vi "Register Image Event.vi"(8 "Error In":errorcluster, 10 "User Event":T1, 11 "Image Object":T2={"Device ID"=0, "Memeroy ID"=0, "Image Parameters"={"Channel Order"=enum."CL_LUMINANCE (Grayscale)", "Dimension"={"Depth"=1, "Height"=1, "Width"=1}, "Data Type"=enum."32f", "Offset"={"X"=0, "Y"=0, "Z"=0}}} {"Image Parameters"."Dimension"."Width" min=1; "Image Parameters"."Dimension"."Height" min=1; "Image Parameters"."Dimension"."Depth" min=1}) -> (0 "Error Out":errorcluster, 2 "User Event Out":T1, 3 "Memory Object Out":T2={"Device ID"=0, "Memeroy ID"=0, "Image Parameters"={"Channel Order"=enum."CL_LUMINANCE (Grayscale)", "Dimension"={"Depth"=1, "Height"=1, "Width"=1}, "Data Type"=enum."32f", "Offset"={"X"=0, "Y"=0, "Z"=0}}} {"Image Parameters"."Dimension"."Width" min=1; "Image Parameters"."Dimension"."Height" min=1; "Image Parameters"."Dimension"."Depth" min=1})   [LabVIEW 2012, in "OpenCLV x64.lvlib"]
doc: "Registers an image user event using a Boolean Labview User Event. Once an image has been registered with a Labview User Event, it can be read and written to asynchronously (non-blocking) to allow other tasks to be performed by the program including user inputs to the front panel.\n\nThis is useful when copying very large datasets to the device."
uses:
  OpenCLV x64.lvlib
  Controls/Image Object.ctl
  Controls/Device ID.ctl
  Controls/Memory ID.ctl
  Controls/Image Parameters.ctl
  Images/Channel Order.ctl
  User Controls/Array Dimensions.ctl
  Images/Data Type.ctl
  User Controls/Offset.ctl
  Controls/User Event.ctl
  Error Checking/Add Error Functional Global.vi
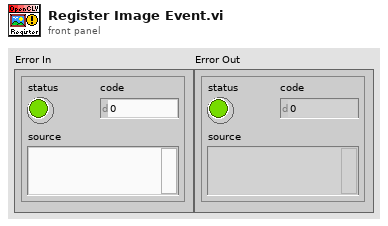
[diagram p1: front panel]
types:
  T1 = typedef "OpenCLV x64.lvlib/User Event.ctl" = refnum<user-event>
  T2 = typedef "OpenCLV x64.lvlib/Image Object.ctl" = cluster{"Device ID":T3, "Memeroy ID":T4, "Image Parameters":T5}
  T3 = typedef "OpenCLV x64.lvlib/Device ID.ctl" = u64
  T4 = typedef "OpenCLV x64.lvlib/Memory ID.ctl" = u64
  T5 = typedef "OpenCLV x64.lvlib/Image Parameters.ctl" = cluster{"Channel Order":T6, "Dimension":T7, "Data Type":T8, "Offset":T9}
  T6 = typedef "OpenCLV x64.lvlib/Channel Order.ctl" = enum16{"CL_LUMINANCE (Grayscale)", "CL_INTENSITY (Opacity)", "CL_RGBA", "CL_ARGB", "CL_BGRA", "CL_RG", "CL_RA", "CL_R", "CL_A"}
  T7 = typedef "Array Dimensions.ctl" = cluster{"Depth":u64, "Height":u64, "Width":u64}
  T8 = typedef "OpenCLV x64.lvlib/Data Type.ctl" = enum16{"32f", "u8", "u16", "u32", "i8", "i16", "i32"}
  T9 = typedef "Offset.ctl" = cluster{"X":u64, "Y":u64, "Z":u64}
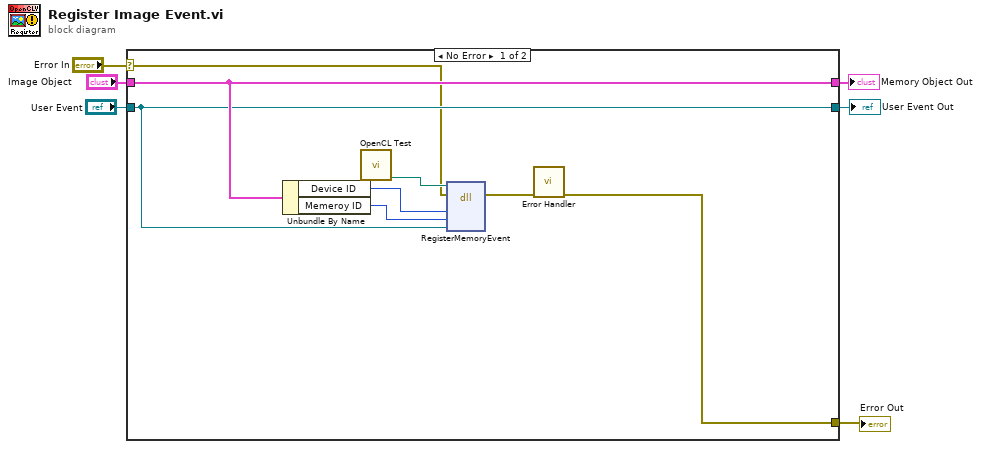
[diagram p0: block diagram]
diagram:
  n1 = case shown="No Error" "Error In" {
    selector: "Error In" -> [w7 w17]
    tunnel: [w8 w17] -> w5
    tunnel: "Image Object" -> [w11 w15]
    tunnel: "User Event" -> [w10 w16]
    tunnel: [w11 w15] -> w3
    tunnel: [w10 w16] -> w1
    frame No Error {
      n2 = Unbundle By Name(w11) -> ("Device ID"=w12:T3, "Memeroy ID"=w13:T4)
      n3 = call "OpenCL Test.vi"() -> ("DLL To Use"=w14:path)  [unwired: 11 in]
      n4 = dll-call lib="D:/OpenCLV/trunk/OpenCLV_x64_1.0/OpenCLV_x64.dll" fn="RegisterMemoryEvent"(path in=w14, error in=w7, "Device"=w12, "Memory"=w13, "Labview Event"=w10) -> (error out=w9:errorcluster)  [unwired: 5 in, 1 out]
      n5 = call-poly "Error Handler.vi"("Error In"=w9) -> ("Error Out"=w8:errorcluster)  [unwired: 10 in]
    }
    frame Error {
    }
  }
  "Error Out" <- w5
  "Memory Object Out" <- w3
  "User Event Out" <- w1
